vi "Get_mod_dates.vi"(3 "error in (no error)":errorcluster) -> (0 "error out":errorcluster, 2 "Output string":string)   [LabVIEW 2010]
doc: "Gathers information about all VIs currently in memory.\n\nFor each VI, it produces this information:\n1) The path to the VI's file.\n2) The size of the data space attached to the VI's front panel. A re-entrant VI has a data space for each usage of the VI. Therefore, this number is not a true reflection of the amount of data a VI is responsible for.\n3&4) The size of the VI's front panel and the number of objects in it; both are zero if the front panel is not currently in memory.\n5&6) Same as above for the block diagram\n7) size of the code genereated for this VI.\n8) the VI's description.\n9) The VI's handle.\n10) the indices into the raw data array of this VI's callers\n11) the indices into the raw data array of this VI's callees (subVIs)."
panel:
  out "App.Version":string
  out "Results":string[][](table)
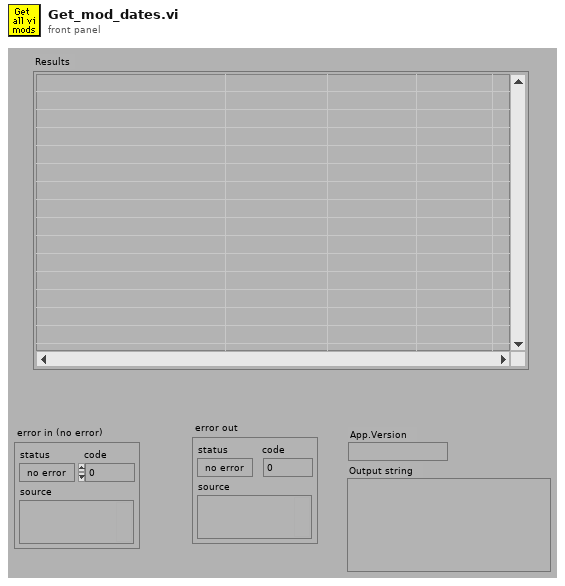
[diagram p1: front panel]
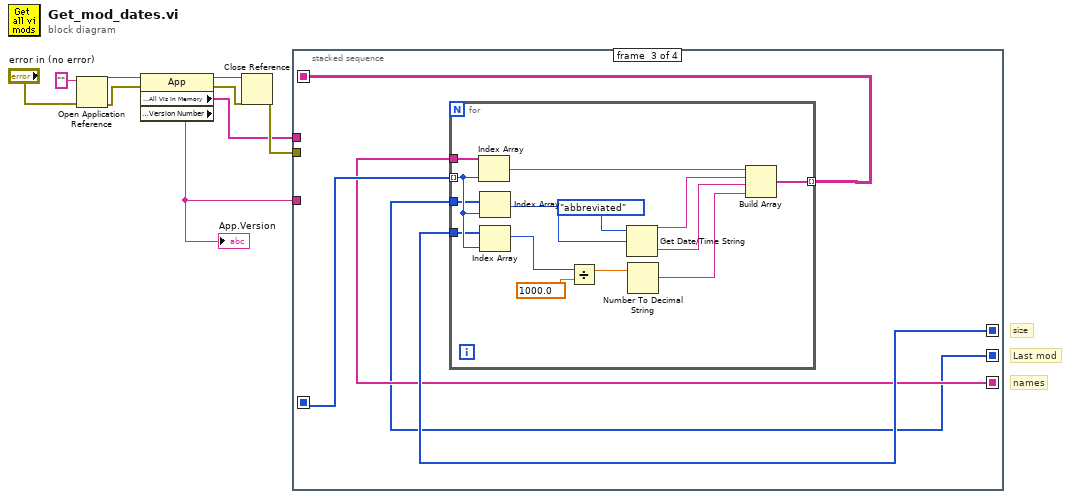
[diagram p0: block diagram]
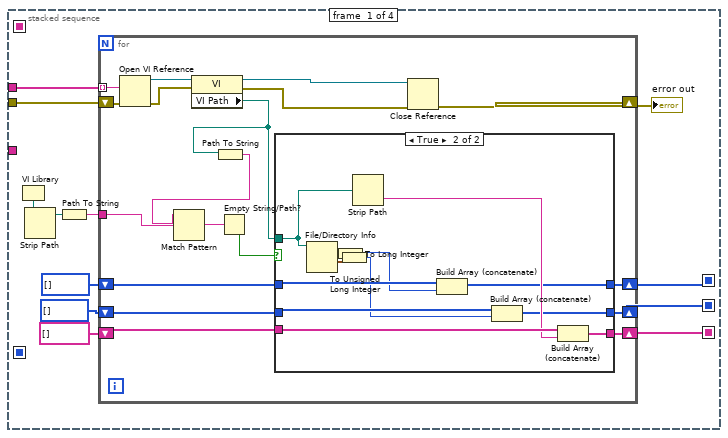
[diagram p2: hidden frame]
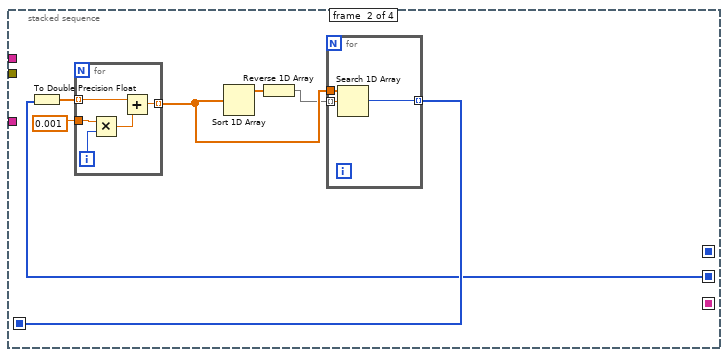
[diagram p4: hidden frame]
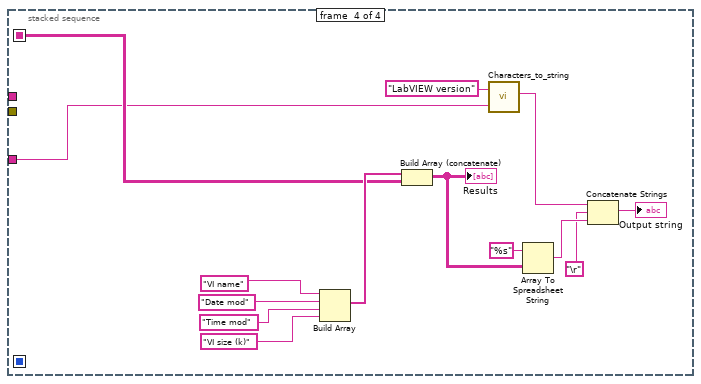
[diagram p5: hidden frame]
diagram:
  # "names"
  # "Last mod"
  # "size"
  n1 = Open Application Reference(8:"error in (no error)", 11:"" ("machine name (\"\":  open local reference)")) -> (0:w8:errorcluster, 3:w9:refnum<vi>)  [unwired: 2 out]
  n2 = property class="App"(reference=w9, error in=w8) -> (reference out=w7:refnum<vi>, error out=w6:errorcluster, "Application:All VIs In Memory"=w2:string[], "Application:Version Number"=w1:string)
  "App.Version" <- w1
  n3 = Close Reference(reference=w7, error in (no error)=w6) -> (error out=w5:errorcluster)
  n4 = stacked-sequence {
    seq-local: [w12 _ _ _] -> [_ _ w73 _]
    seq-local: [w11 _ _ _] -> [_ w57 w71 _]
    seq-local: [w10 _ _ _] -> [_ _ w72 _]
    seq-local: [_ w58 _ _] -> [_ _ w74 _]
    seq-local: [_ _ w70 _] -> [_ _ _ w97]
    tunnel: w5 -> [w21 _ _ _]
    tunnel: w2 -> [w13 _ _ _]
    tunnel: w1 -> [_ _ _ w93]
    frame #0 {
      n5 = VI Library() -> (path=w19:path)
      n6 = Strip Path(path=w19) -> (stripped path=w18:path)  [unwired: 1 out]
      n7 = Path To String(path=w18) -> (string=w17:string)
      n8 = for {
        tunnel: w13 -> [w38] mode=indexing
        shift-right: [w36] -> w20
        shift-left: w21 -> [w37]
        shift-right: [w29] -> w10
        shift-left: string[] [] -> [w30]
        shift-right: [w22] -> w11
        shift-left: u32[] [] -> [w28]
        tunnel: w17 -> [w25]
        shift-right: [w24] -> w12
        shift-left: i32[] [] -> [w23]
        n9 = Open VI Reference(vi path=w38, error in (no error)=w37) -> (vi reference=w33:refnum<vi>, error out=w39:errorcluster)  [unwired: 4 out]
        n10 = property class="VI"(reference=w33, error in=w39) -> (reference out=w34:refnum<vi>, error out=w35:errorcluster, "VI Path"=w26:path)
        n11 = Path To String(path=w26) -> (string=w27:string)
        n12 = Match Pattern(string=w27, regular expression=w25) -> (match substring=w32:string)  [unwired: 4 out]
        n13 = Empty String/Path?(string/path=w32) -> (empty?=w31:bool)
        n14 = case shown="True" w31 {
          tunnel: w26 -> [_ w52]
          tunnel: w30 -> [w42 w54]
          tunnel: [w42 w53] -> w29
          tunnel: w28 -> [w40 w49]
          tunnel: [w41 w47] -> w24
          tunnel: w23 -> [w41 w50]
          tunnel: [w40 w48] -> w22
          frame False {
          }
          frame True {
            n15 = File/Directory Info(path=w52) -> (size=w43:i64, last mod=w44:timestamp)  [unwired: 1 in, 5 out]
            n16 = To Long Integer(number=w43) -> (32bit integer=w46:i32)
            n17 = To Unsigned Long Integer(number=w44) -> (unsigned 32bit integer=w45:u32)
            n18 = Strip Path(path=w52) -> (name=w51:string)  [unwired: 1 out]
            n19 = Build Array (concatenate)(w50, w46) -> (w47:i32[])
            n20 = Build Array (concatenate)(w49, w45) -> (w48:u32[])
            n21 = Build Array (concatenate)(w54, w51) -> (w53:string[])
          }
        }
        n22 = Close Reference(reference=w34, error in (no error)=w35) -> (error out=w36:errorcluster)
      }
      "error out" <- w20
    }
    frame #1 {
      n23 = To Double Precision Float(number=w57) -> (double precision float=w60:dbl[])
      n24 = for {
        tunnel: w60 -> [w66] mode=indexing
        tunnel: 0.001 -> [w63]
        tunnel: [w62] -> w56 mode=indexing
        i -> [w64]
        n25 = Multiply(x=w63, y=w64) -> (x*y=w65:dbl)
        n26 = Add(x=w66, y=w65) -> (x+y=w62:dbl)
      }
      n27 = Sort 1D Array(array=w56) -> (sorted array=w61:dbl[])
      n28 = Reverse 1D Array(array=w61) -> (reversed array=w55:dbl[])
      n29 = for {
        tunnel: w56 -> [w69]
        tunnel: w55 -> [w68] mode=indexing
        tunnel: [w67] -> w58 mode=indexing
        n30 = Search 1D Array(1D array=w69, element=w68) -> (index of element=w67:i32)  [unwired: 1 out]
      }
    }
    frame #2 {
      n31 = for {
        tunnel: w74 -> [w87] mode=indexing
        tunnel: w72 -> [w88]
        tunnel: w71 -> [w84]
        tunnel: w73 -> [w83]
        tunnel: [w79] -> w70 mode=indexing
        n32 = Index Array(array=w88, index=w87) -> (element=w85:string)
        n33 = Index Array(array=w84, index=w87) -> (element=w75:u32)
        n34 = Index Array(array=w83, index=w87) -> (element=w78:i32)
        n35 = Divide(x=w78, y=1000.0) -> (x/y=w76:dbl)
        n36 = Get Date/Time String(date format (0)=enum16{"short", "long", "abbreviated"}."abbreviated", seconds (now)=w75) -> (date string=w82:string, time string=w81:string)  [unwired: 1 out]
        n37 = Number To Decimal String(number=w76) -> (decimal integer string=w80:string)  [unwired: 1 out]
        n38 = Build Array(w85, w82, w81, w80) -> (w79:string[])
      }
    }
    frame #3 {
      n39 = Build Array("VI name", "Date mod", "Time mod", "VI size (k)") -> (w98:string[])
      n40 = Build Array (concatenate)(w98, w97) -> (w95:string[][])
      "Results" <- w95
      n41 = call "Characters_to_string.vi"("Characters to write"=w93, "Label for characters"="LabVIEW version") -> ("Output string"=w91:string)
      n42 = Array To Spreadsheet String(array=w95, 3:"%s" ("format string")) -> (spreadsheet string=w94:string)  [unwired: 1 out]
      n43 = Concatenate Strings(w91, "\r", w94) -> (→"Output string":string)
    }
  }
